vi "231107_Nikon_Control.vi"() -> ()   [LabVIEW 2014]
panel:
  in  "Cluster commandes":T1={"Dia lamp"=TRUE, "Dia lamp intensity"=1689.1304347826087, "Objective"=2, "Light path"=2, "Z pos (µm)"=335593} {"Z pos (µm)" min=0 max=990000 step=100 scale=0.0..990000.0; "Light path" items=["1- Eyepiece"=1, "2- Right"=2, "3- Left + Eyepiece"=3, "4- Left"=4]; "Objective" items=["1- Target"=1, "2- PLAN APO 100X 1,45 Oil"=2, "3- Empty"=3, "4- Empty"=4, "5- Empty"=5, "6- Empty"=6]; "Dia lamp intensity" scale=0.0..2100.0}
  out "Cluster µscope":T2
  in  "stop":bool
  in  "NikonTi2AxLib.INikonTi2AxMicroscope":refnum<k7>
  out "error out":errorcluster={"status"=TRUE, "code"=-9, "source"="Exception occured in Nikon.Ti2.Microscope.1: Failed in 231026_NikonTi2_Indicators_v2.vi"} caption="sortie d'erreur"
  in  "error in":errorcluster caption="entrée d'erreur"
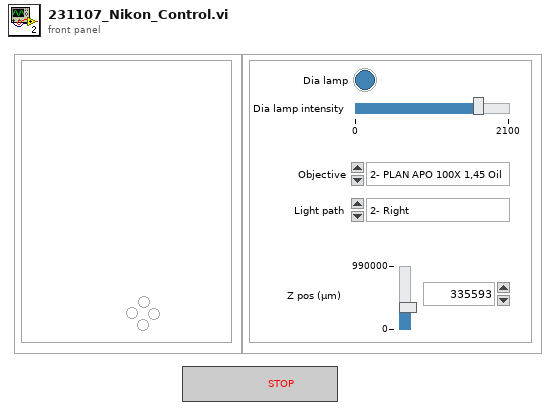
[diagram p1: front panel]
types:
  T1 = cluster{"Dia lamp":bool, "Dia lamp intensity":dbl, "Objective":i32, "Light path":u32, "Z pos (µm)":i32}
  T2 = cluster{"Eyepiece":bool, "Right":bool, "Left + Eyepiece":bool, "Left":bool}
  T3 = cluster{"iNOSEPIECE":i32, "iLIGHTPATH":i32, "iDIA_LAMP_Switch":i32, "iDIA_LAMP_Pos":i32, "iZPOSITION":i32, "iPFS_SWITCH":i32, "iPFS_STATUS":i32, "iPFS_OFFSET":i32}
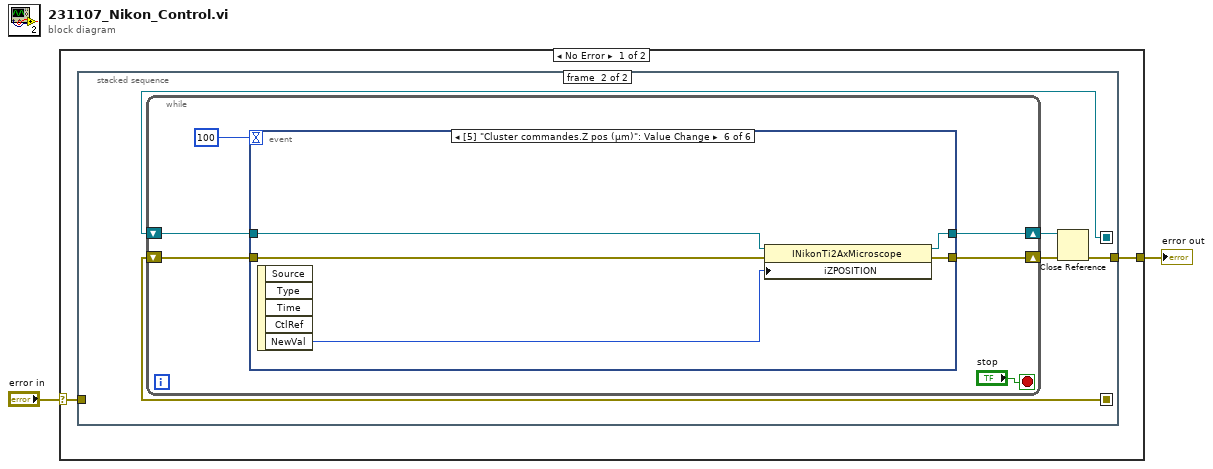
[diagram p0: block diagram]
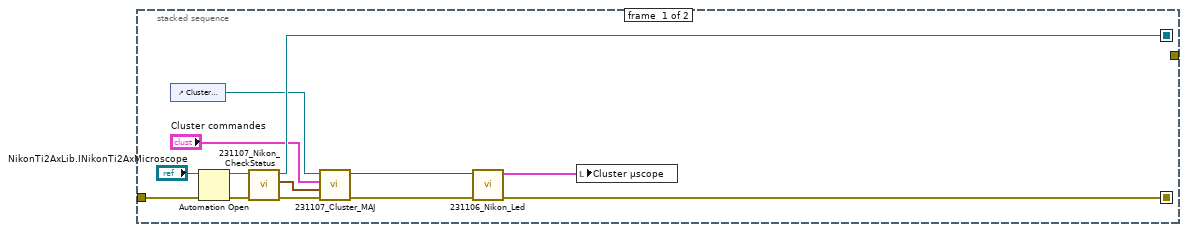
[diagram p2: hidden frame]
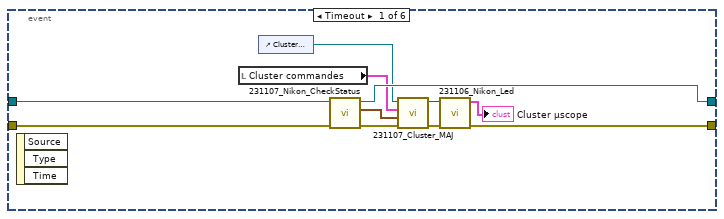
[diagram p3: hidden frame]
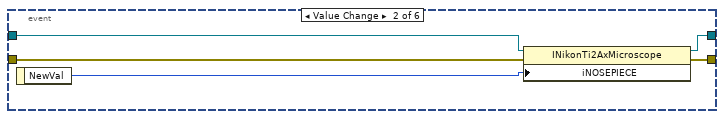
[diagram p4: hidden frame]
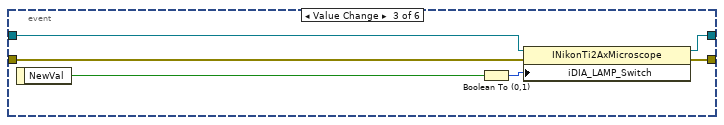
[diagram p5: hidden frame]
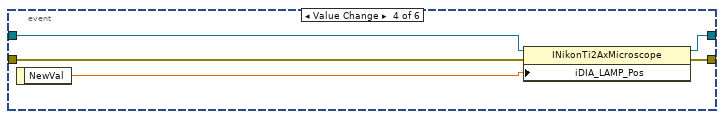
[diagram p6: hidden frame]
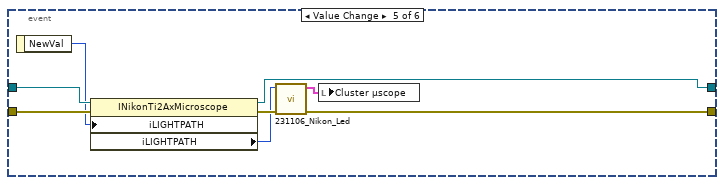
[diagram p7: hidden frame]
diagram:
  n1 = case shown="No Error" "error in" {
    selector: "error in" -> [w4 w69]
    tunnel: [w3 w69] -> w1
    frame No Error {
      n2 = stacked-sequence {
        seq-local: [w13 _] -> [_ w22]
        seq-local: [w6 _] -> [_ w18]
        tunnel: w4 -> [w14 _]
        tunnel: [_ w19] -> w3
        frame #0 {
          n3 = control-ref of="Cluster commandes"() -> (w5:refnum<vi>)
          n4 = Automation Open(error in (no error)=w14, Automation Refnum="NikonTi2AxLib.INikonTi2AxMicroscope") -> (Automation Refnum=w16:refnum<k7>, error out=w15:errorcluster)  [unwired: 2 in]
          n5 = call "231107_Nikon_CheckStatus.vi"("error in"=w15, "NikonTi2AxLib.INikonTi2AxMicroscope"=w16) -> ("error out"=w8:errorcluster, "Nikon status cluster"=w12:T3, "reference out"=w13:refnum<k7>)  [unwired: 7 in]
          n6 = call "231107_Cluster_MAJ.vi"("error in (no error)"=w8, "Nikon status cluster"=w12, 10:"Cluster commandes"="Cluster commandes", 11:"Cluster commandes"=w5) -> ("error out"=w7:errorcluster, "iLIGHTPATH"=w9:i32)  [unwired: 6 in]
          n7 = call "231106_Nikon_Led.vi"("error in"=w7, "Light path"=w9) -> ("error out"=w6:errorcluster, "Cluster µscope"=w11:T2)  [unwired: 8 in]
          n8 = local write "Cluster µscope"(w11) -> ()
        }
        frame #1 {
          n9 = while {
            shift-right: [w23] -> w20
            shift-left: w18 -> [w28]
            shift-right: [w24] -> w21
            shift-left: w22 -> [w25]
            stop <- "stop" stop-if-true
            n10 = event shown="[5] \"Cluster commandes.Z pos (µm)\": Value Change" {
              selector: _ -> [_ _ _ _ _ _]
              dyn-events: _ -> [_ _ _ _ _ _]
              timeout: 100 -> [_ _ _ _ _ _]
              tunnel: [w36 w41 w47 w52 w60 w67] -> w23
              tunnel: w28 -> [w39 w43 w49 w54 w61 w65]
              tunnel: w25 -> [w38 w44 w50 w55 w62 w66]
              tunnel: [w37 w42 w48 w53 w63 w68] -> w24
              event Timeout {
                n11 = event-data() -> ()  [unwired: 1 in, 3 out]
                n12 = local read "Cluster commandes"() -> (w30:T1)
                n13 = control-ref of="Cluster commandes"() -> (w29:refnum<vi>)
                n14 = call "231107_Nikon_CheckStatus.vi"("error in"=w39, "NikonTi2AxLib.INikonTi2AxMicroscope"=w38) -> ("error out"=w33:errorcluster, "Nikon status cluster"=w34:T3, "reference out"=w37:refnum<k7>)  [unwired: 7 in]
                n15 = call "231107_Cluster_MAJ.vi"("error in (no error)"=w33, "Nikon status cluster"=w34, 10:"Cluster commandes"=w30, 11:"Cluster commandes"=w29) -> ("error out"=w32:errorcluster, "iLIGHTPATH"=w31:i32)  [unwired: 6 in]
                n16 = call "231106_Nikon_Led.vi"("error in"=w32, "Light path"=w31) -> ("error out"=w36:errorcluster, "Cluster µscope"=→"Cluster µscope":T2)  [unwired: 8 in]
              }
              event "Cluster commandes.Objective": Value Change {
                n17 = event-data() -> ("NewVal"=w40:i32)  [unwired: 1 in]
                n18 = property class="INikonTi2AxMicroscope"(reference=w44, error in=w43, "iNOSEPIECE"=w40) -> (reference out=w42:refnum<k7>, error out=w41:errorcluster)
              }
              event "Cluster commandes.Dia lamp": Value Change {
                n19 = event-data() -> ("NewVal"=w46:bool)  [unwired: 1 in]
                n20 = Boolean To (0,1)(Boolean=w46) -> (0, 1=w45:i16)
                n21 = property class="INikonTi2AxMicroscope"(reference=w50, error in=w49, "iDIA_LAMP_Switch"=w45) -> (reference out=w48:refnum<k7>, error out=w47:errorcluster)
              }
              event "Cluster commandes.Dia lamp intensity": Value Change {
                n22 = event-data() -> ("NewVal"=w51:dbl)  [unwired: 1 in]
                n23 = property class="INikonTi2AxMicroscope"(reference=w55, error in=w54, "iDIA_LAMP_Pos"=w51) -> (reference out=w53:refnum<k7>, error out=w52:errorcluster)
              }
              event "Cluster commandes.Light path": Value Change {
                n24 = event-data() -> ("NewVal"=w57:u32)  [unwired: 1 in]
                n25 = property class="INikonTi2AxMicroscope"(reference=w62, error in=w61, "iLIGHTPATH"=w57) -> (reference out=w63:refnum<k7>, error out=w59:errorcluster, "iLIGHTPATH"=w58:i32)
                n26 = call "231106_Nikon_Led.vi"("error in"=w59, "Light path"=w58) -> ("error out"=w60:errorcluster, "Cluster µscope"=w56:T2)  [unwired: 8 in]
                n27 = local write "Cluster µscope"(w56) -> ()
              }
              event "Cluster commandes.Z pos (µm)": Value Change {
                n28 = event-data() -> ("NewVal"=w64:i32)  [unwired: 1 in, 4 out]
                n29 = property class="INikonTi2AxMicroscope"(reference=w66, error in=w65, "iZPOSITION"=w64) -> (reference out=w68:refnum<k7>, error out=w67:errorcluster)
              }
            }
          }
          n30 = Close Reference(reference=w21, error in (no error)=w20) -> (error out=w19:errorcluster)
        }
      }
    }
    frame Error {
    }
  }
  "error out" <- w1
